vi "Transmitter.vi"() -> ()   [LabVIEW 2013]
uses:
  <vilib>/sound2/lvsound2.llb/Sound File Info (path).vi
  <vilib>/sound2/lvsound2.llb/Sound File Read Open.vi
  <vilib>/sound2/lvsound2.llb/Sound File Read (DBL).vi
  <vilib>/Analysis/NI_AALPro.lvlib
  <vilib>/Analysis/2dsp.llb/Rational Resample (single channel, DBL).vi
  <instrlib>/niUSRP/niUSRP Write Tx Data (CDB).vi
  <vilib>/Analysis/NI_AALBase.lvlib
  <vilib>/Analysis/3filter.llb/IIR Filter (DBL).vi
  <vilib>/express/express analysis/Spectral/Block/exnSpectralBlock spectral measurements RMS poly.vi
  <vilib>/express/express analysis/Spectral/Block/exnSpectralBlock spectral measurements RMS WFM.vi
  <vilib>/express/express analysis/Spectral/XNode/ExpressSpectralMeasurementsBlockNode.xnode
panel:
  out "coerced IQ rate":dbl=200000.0 format="%#_6p"
  in  "IQ rate":dbl(slide)=200000.0 scale=0.0..10.0
  in  "IP":refnum<k15>="192.168.10.2"
  in  "Path":path=path "E:/TianyangChen/ComProject_I/LoveUSRP/International.wav"
  in  "Stop":bool
  out "Error Out":errorcluster
  out "Spectrum(FFT)":cluster{"f0":dbl, "df":dbl, "magnitude":dbl[]}(graph)
  out "Constellatiom":cluster{dbl[], dbl[]}(graph)
  out "Waveform":waveform(dbl)(graph)
  in  "FM deviation":dbl=50.0 format="%#_6f"
  in  "active antenna":string="TX1"
  out "coerced gain":dbl format="%#_6p"
  out "coerced carrier frequency":dbl=2400000000.0 format="%#_6p"
  in  "number of samples":i32=22050
  in  "gain":dbl format="%#_6f"
  in  "carrier frequency":dbl=3500000000.0 format="%#_6p"
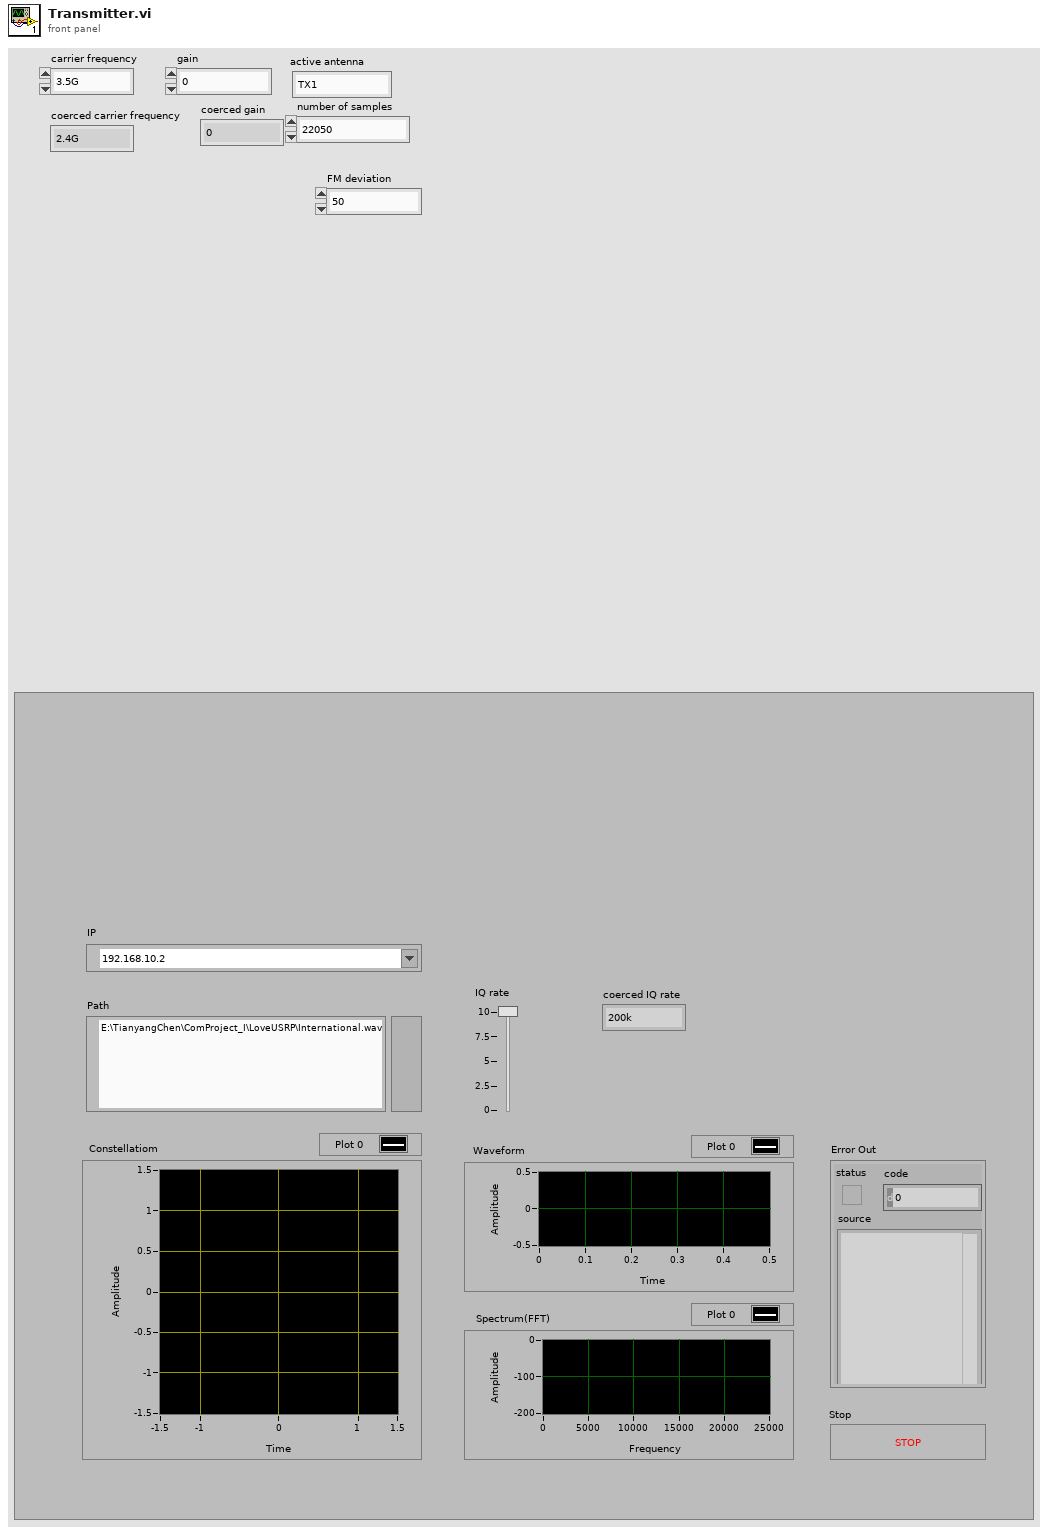
[diagram p1: front panel]
types:
  T1 = typedef "Sound Data Format.ctl" = cluster{"sample rate (S/s)":dbl, "number of channels":i32, "bits per sample":i32}
  T2 = typedef "Sound File Refnum.ctl" = refnum<file>
  T3 = cluster{"averaging mode":u16, "weighting mode":u16, "number of averages":u32}
  T4 = cluster{"dB On (F)":bool, "unwrap phase (F)":bool, "convert to degree (F)":bool}
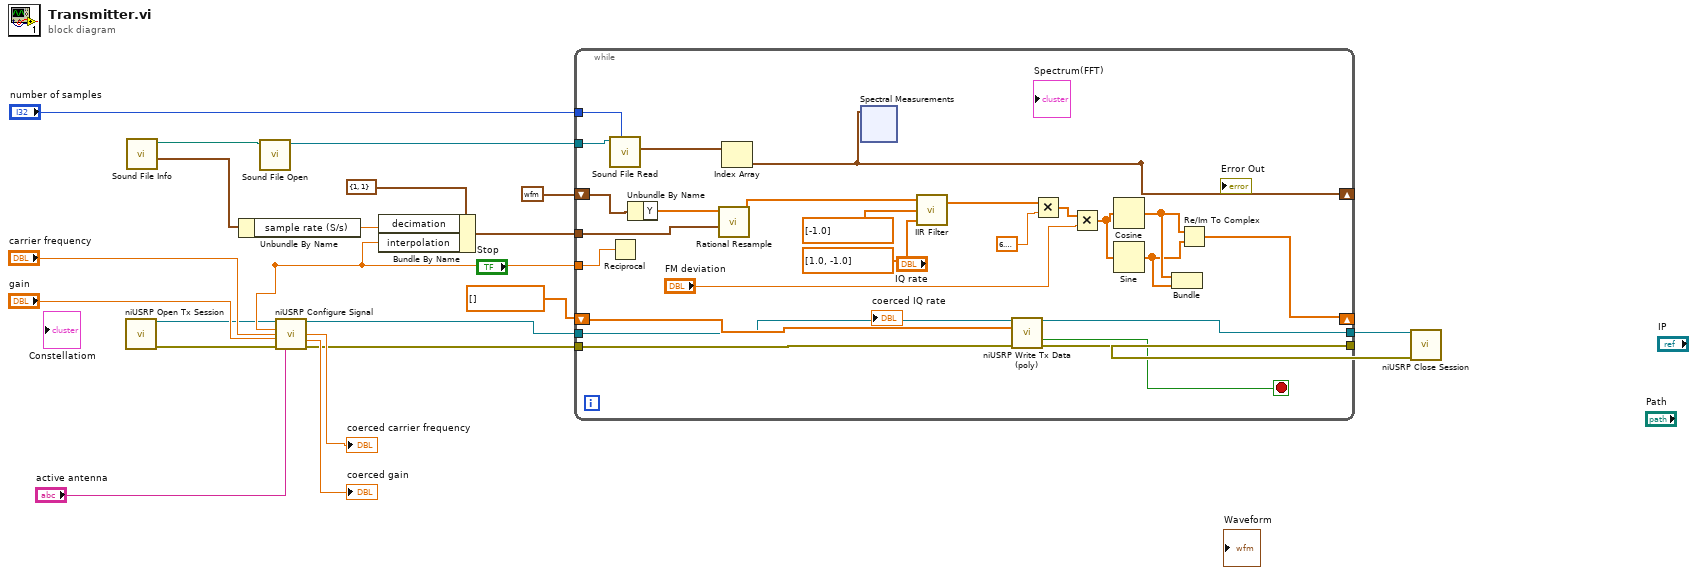
[diagram p0: block diagram]
diagram:
  n1 = call <instrlib>:"niUSRP Open Tx Session.vi"() -> ("device names"=w2:refnum<k15>, "session handle out"=w1:refnum<k15>, "error out"=w21:errorcluster)  [unwired: 13 in]
  n2 = call-poly <vilib>:"Sound File Info.vi"() -> ("sound format"=w15:T1, "path out"=w25:path, "path"=w23:path)  [unwired: 7 in, 2 out]
  n3 = Unbundle By Name(w15) -> ("sample rate (S/s)"=w14:dbl)
  n4 = call-poly <vilib>:"Sound File Open.vi"("path"=w25) -> ("sound file refnum"=w24:T2)  [unwired: 9 in, 1 out]
  n5 = call <instrlib>:"niUSRP Configure Signal.vi"("session handle"=w1, "IQ rate"=w3, "carrier frequency"="carrier frequency", "gain"="gain", "error in (no error)"=w21, "active antenna"="active antenna") -> ("session handle out"=w13:refnum<k15>, "coerced IQ rate"=w19:dbl, "coerced carrier frequency"=→"coerced carrier frequency":dbl, "coerced gain"=→"coerced gain":dbl, "error out"=w10:errorcluster)  [unwired: 5 in]
  n6 = Bundle By Name(cluster=cluster{"interpolation":i32, "decimation":i32} {"interpolation"=1, "decimation"=1} ("input cluster"), "decimation"=w14, "interpolation"=w3) -> (w6:cluster{"interpolation":i32, "decimation":i32})
  n7 = while {
    tunnel: w24 -> [w52]
    tunnel: "number of samples" -> [w51]
    shift-right: [w26] -> _
    shift-left: waveform(dbl) {"t0"=timestamp(0 s since 1904-01-01), "dt"=1.0, "Y"=[]} ("waveform") -> [w49]
    shift-right: [w41] -> _
    shift-left: cdb[] [] ("data") -> [w40]
    tunnel: w13 -> [w39]
    tunnel: [w38] -> w12
    tunnel: [w37] -> w11
    tunnel: w10 -> [w36]
    tunnel: w6 -> [w35]
    tunnel: [w32] -> w3
    stop <- w34 stop-if-true
    n8 = call-poly <vilib>:"Sound File Read.vi"("number of samples/ch (-1: all)"=w51, "sound file refnum"=w52) -> ("data"=w50:waveform(dbl)[])  [unwired: 5 in, 4 out]
    n9 = Reciprocal(x=w32) -> ()  [unwired: 1 out]
    n10 = Unbundle By Name(w49) -> ("Y"=w48:dbl[])
    n11 = call-poly <vilib>:"Rational Resample.vi"("resample factor"=w35, "X"=w48) -> ("Y"=w31:dbl[])  [unwired: 7 in, 2 out]
    n12 = Index Array(array=w50) -> (element=w26:waveform(dbl))  [unwired: 1 in]
    n13 = xnode "Spectral Measurements"("Signals"=w26) -> ("FFT - (RMS)"=w27:cluster{"f0":dbl, "df":dbl, "magnitude":dbl[]})  [unwired: 1 in, 2 out]
    n14 = call-poly <vilib>:"IIR Filter.vi"("Forward Coefficients"=dbl[] [1.0, -1.0], "Reverse Coefficients"=dbl[] [-1.0], "X"=w31) -> ("Filtered X"=w30:dbl[])  [unwired: 1 in, 1 out]
    n15 = call-poly <instrlib>:"niUSRP Write Tx Data (poly).vi"("session handle"=w39, "data"=w40, "error in (no error)"=w36) -> ("session handle out"=w38:refnum<k15>, "end of data?"=w34:bool, "error out"=w37:errorcluster)  [unwired: 10 in]
    n16 = Multiply(x=w30, y=6.283185307179586) -> (x*y=w47:dbl[])
    n17 = Multiply(x=w47, y="FM deviation") -> (x*y=w44:dbl[])
    n18 = Cosine(x=w44) -> (cos(x)=w43:dbl[])
    n19 = Sine(x=w44) -> (sin(x)=w42:dbl[])
    n20 = Bundle(w43, w42) -> (w33:cluster{dbl[], dbl[]})  [unwired: 1 in]
    n21 = Re/Im To Complex(1:w42, 2:w43) -> (0:w41:cdb[])
  }
  n22 = call <instrlib>:"niUSRP Close Session.vi"("session handle"=w12, "error in (no error)"=w11) -> ("error out"=w9:errorcluster)  [unwired: 13 in]
